vi "Create.vi"() -> (8 "Gate":refnum<class "Gate.lvclass">)   [LabVIEW 2020, in "Gate.lvclass"]
uses:
  Gate.lvclass
  Shape.ctl
  Gate.lvclass/Gate.ctl
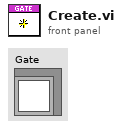
[diagram p1: front panel]
types:
  T1 = typedef "Gate.lvclass/Shape.ctl" = enum16{"OFF", "Rectangle", "Sine-squared", "Trapezoid"}
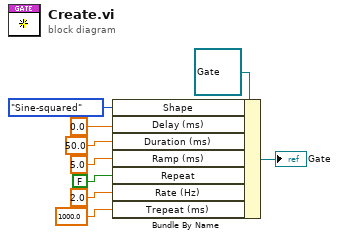
[diagram p0: block diagram]
diagram:
  n1 = Bundle By Name(cluster=refnum<class "Gate.lvclass"> refnum ("Gate"), "Shape"=Shape."Sine-squared" ("Serialized.Shape"), "Delay (ms)"=0.0 ("Serialized.Delay (ms)"), "Duration (ms)"=50.0 ("Serialized.Duration (ms)"), "Ramp (ms)"=5.0 ("Serialized.Ramp (ms)"), "Repeat"=FALSE ("Serialized.Repeat"), "Rate (Hz)"=2.0 ("Serialized.Rate (Hz)"), "Trepeat (ms)"=1000.0 ("Serialized.Trepeat (ms)")) -> (→"Gate":refnum<class "Gate.lvclass">)
